vi "load station config.vi"(8 "error in":errorcluster, 11 "station config file path":path=path "c:/Labview Code/System/station config.ini") -> (0 "error out":errorcluster, 2 "Line Name":string="TP10 - All Stations Status", 3 "all satation cluster":T1[](array[typedef]) {"LIN INFO"."NAD" format="%.0x"; "LIN INFO"."ADCS LIN"."HW select" items=["NI-XNET", "NI-CAN"]; "LVDT Status"."LVDT's stored config"."Lower Limit" format="%.2f"; "LVDT Status"."LVDT's stored config"."Upper Limit" format="%.2f"; "Store Data"."Sun Shade Open Force Limits"."Variance" format="%.2g"; "Store Data"."Sun Shade Open Force Limits"."Truncation End" format="%.2g"; "Store Data"."Sun Shade Open Force Limits"."Truncation Start" format="%.2g"; "Store Data"."Sun Shade Open Force Limits"."Avg Max" format="%.2g"; "Store Data"."Sun Shade Open Force Limits"."Avg Min" format="%.2g"; "Store Data"."Sun Shade Open Force Limits"."Overall Max" format="%.2g"; "Store Data"."Sun Shade Open Force Limits"."Overall Min" format="%.2g"; "Store Data"."Sun Shade Close Force Limits"."Variance" format="%.2g"; "Store Data"."Sun Shade Close Force Limits"."Truncation End" format="%.2g"; "Store Data"."Sun Shade Close Force Limits"."Truncation Start" format="%.2g"; "Store Data"."Sun Shade Close Force Limits"."Avg Max" format="%.2g"; "Store Data"."Sun Shade Close Force Limits"."Avg Min" format="%.2g"; "Store Data"."Sun Shade Close Force Limits"."Overall Max" format="%.2g"; "Store Data"."Sun Shade Close Force Limits"."Overall Min" format="%.2g"; "Store Data"."Motion Data Array"."Motion Data Limits"."LIN Msg"."Msg" format="%02x"; "Store Data"."Motion Data Array"."Motion Data Limits"."LIN Msg"."ID" format="%02x"})   [LabVIEW 2018]
uses:
  02.Type Def's/main state cluster.ctl
  02.Type Def's/All Switch Configuration Cluster.ctl
  02.Type Def's/All Motions.ctl
  02.Type Def's/EOL Switch Value Configuration Cluster.ctl
  02.Type Def's/EOL Switch Max Min Check Cluster.ctl
  02.Type Def's/station nvh config.ctl
  02.Type Def's/station rs232 port map.ctl
  02.Type Def's/station ethernet address map.ctl
  02.Type Def's/station paths.ctl
  02.Type Def's/EOL Save Module Test Data Control.ctl
  02.Type Def's/EOL Motion Database Table.ctl
  05.UserVI's/type defs/17x Audit Motion Data Seq Control.ctl
  05.UserVI's/type defs/17x AP Data Type.ctl
  05.UserVI's/type defs/17x Sunshade Limts Seq.ctl
  02.Type Def's/EOL Module Info Control.ctl
  02.Type Def's/station DI map.ctl
  05.UserVI's/type defs/EOL Global Digital Input Control.ctl
  02.Type Def's/control refs.ctl
  02.Type Def's/station motion data indicator.ctl
  02.Type Def's/Screen Motion Data.ctl
  02.Type Def's/Pass Fail Control.ctl
  02.Type Def's/station hmi.ctl
  02.Type Def's/lvdt name val pair.ctl
  02.Type Def's/individual station status.ctl
  02.Type Def's/misc station config.ctl
  05.UserVI's/Lambda Power/power supply types.ctl
  05.UserVI's/type defs/EOL LVDT's Check Controller.ctl
  05.UserVI's/LVDT's/lvdt precision.ctl
  02.Type Def's/sequence state.ctl
  05.UserVI's/sequence/type defs/Sequence Info.ctl
  05.UserVI's/type defs/EOL Part Setup.ctl
  02.Type Def's/All Communication Types.ctl
  05.UserVI's/type defs/Communication with Motors.ctl
  05.UserVI's/type defs/RAP Signal Control.ctl
  05.UserVI's/type defs/EOL Motor Type.ctl
  02.Type Def's/station LIN config.ctl
  03.Inalfa LIN/LIN Device.ctl
  <vilib>/CMC.AME/Inalfa ADCS/Ctl'Def/ADCS_LIN info.ctl
  C:/Program Files (x86)/National Instruments/LabVIEW 2018/vi.lib/CMC.AME/Inalfa TS LIN/TOSUN/TSMaster/bin/Interop.TSMasterAPI.dll
  Program Files (x86)/National Instruments/LabVIEW 2018/vi.lib/CMC.AME/Inalfa TS LIN/TOSUN/TSMaster/bin/Interop.TSMasterAPI.dll
  06.Test Loop/Sub'VIs/Type Def's/Config Info.ctl
  05.UserVI's/file io/ini/type defs/ini entry.ctl
  05.UserVI's/file io/ini/type defs/ini entry types.ctl
  05.UserVI's/file io/ini/type defs/ini entry value.ctl
  05.UserVI's/file io/ini/type defs/ini file actions.ctl
panel:
  # "Sunroof Barcode"
  # "Pallet Number"
  # "Part Type"
  # "Application Status"
  # "Current Step"
  # "Cycle Time"
  # "Pass / Fail"
  # "Shade Close"
  # "Actual Data"
  # "Limits"
  # "Avg Current"
  # "Run Time"
  # "Speed"
  # "Noise Test"
  # "Position"
  # "Shade Open"
  # "Actual Data"
  # "Limits"
  # "Avg Current"
  # "Run Time"
  # "Speed"
  # "Noise Test"
  # "Position"
  # "Vent Close"
  # "Actual Data"
  # "Limits"
  # "Avg Current"
  # "Run Time"
  # "Speed"
  # "Noise Test"
  # "Position"
  # "Vent Open"
  # "Actual Data"
  # "Limits"
  # "Avg Current"
  # "Run Time"
  # "Speed"
  # "Noise Test"
  # "Position"
  # "Slide Close"
  # "Actual Data"
  # "Limits"
  # "Avg Current"
  # "Run Time"
  # "Speed"
  # "Noise Test"
  # "Position"
  # "Slide Open"
  # "Actual Data"
  # "Limits"
  # "Avg Current"
  # "Run Time"
  # "Speed"
  # "Noise Test"
  # "Position"
  # "Min"
  # "N"
  # "Min"
  # "Start"
  # "N"
  # "Max"
  # "N"
  # "Max"
  # "N"
  # "End"
  # "Min"
  # "N"
  # "Min"
  # "Start"
  # "N"
  # "Max"
  # "N"
  # "Max"
  # "N"
  # "End"
  # "Min"
  # "Max"
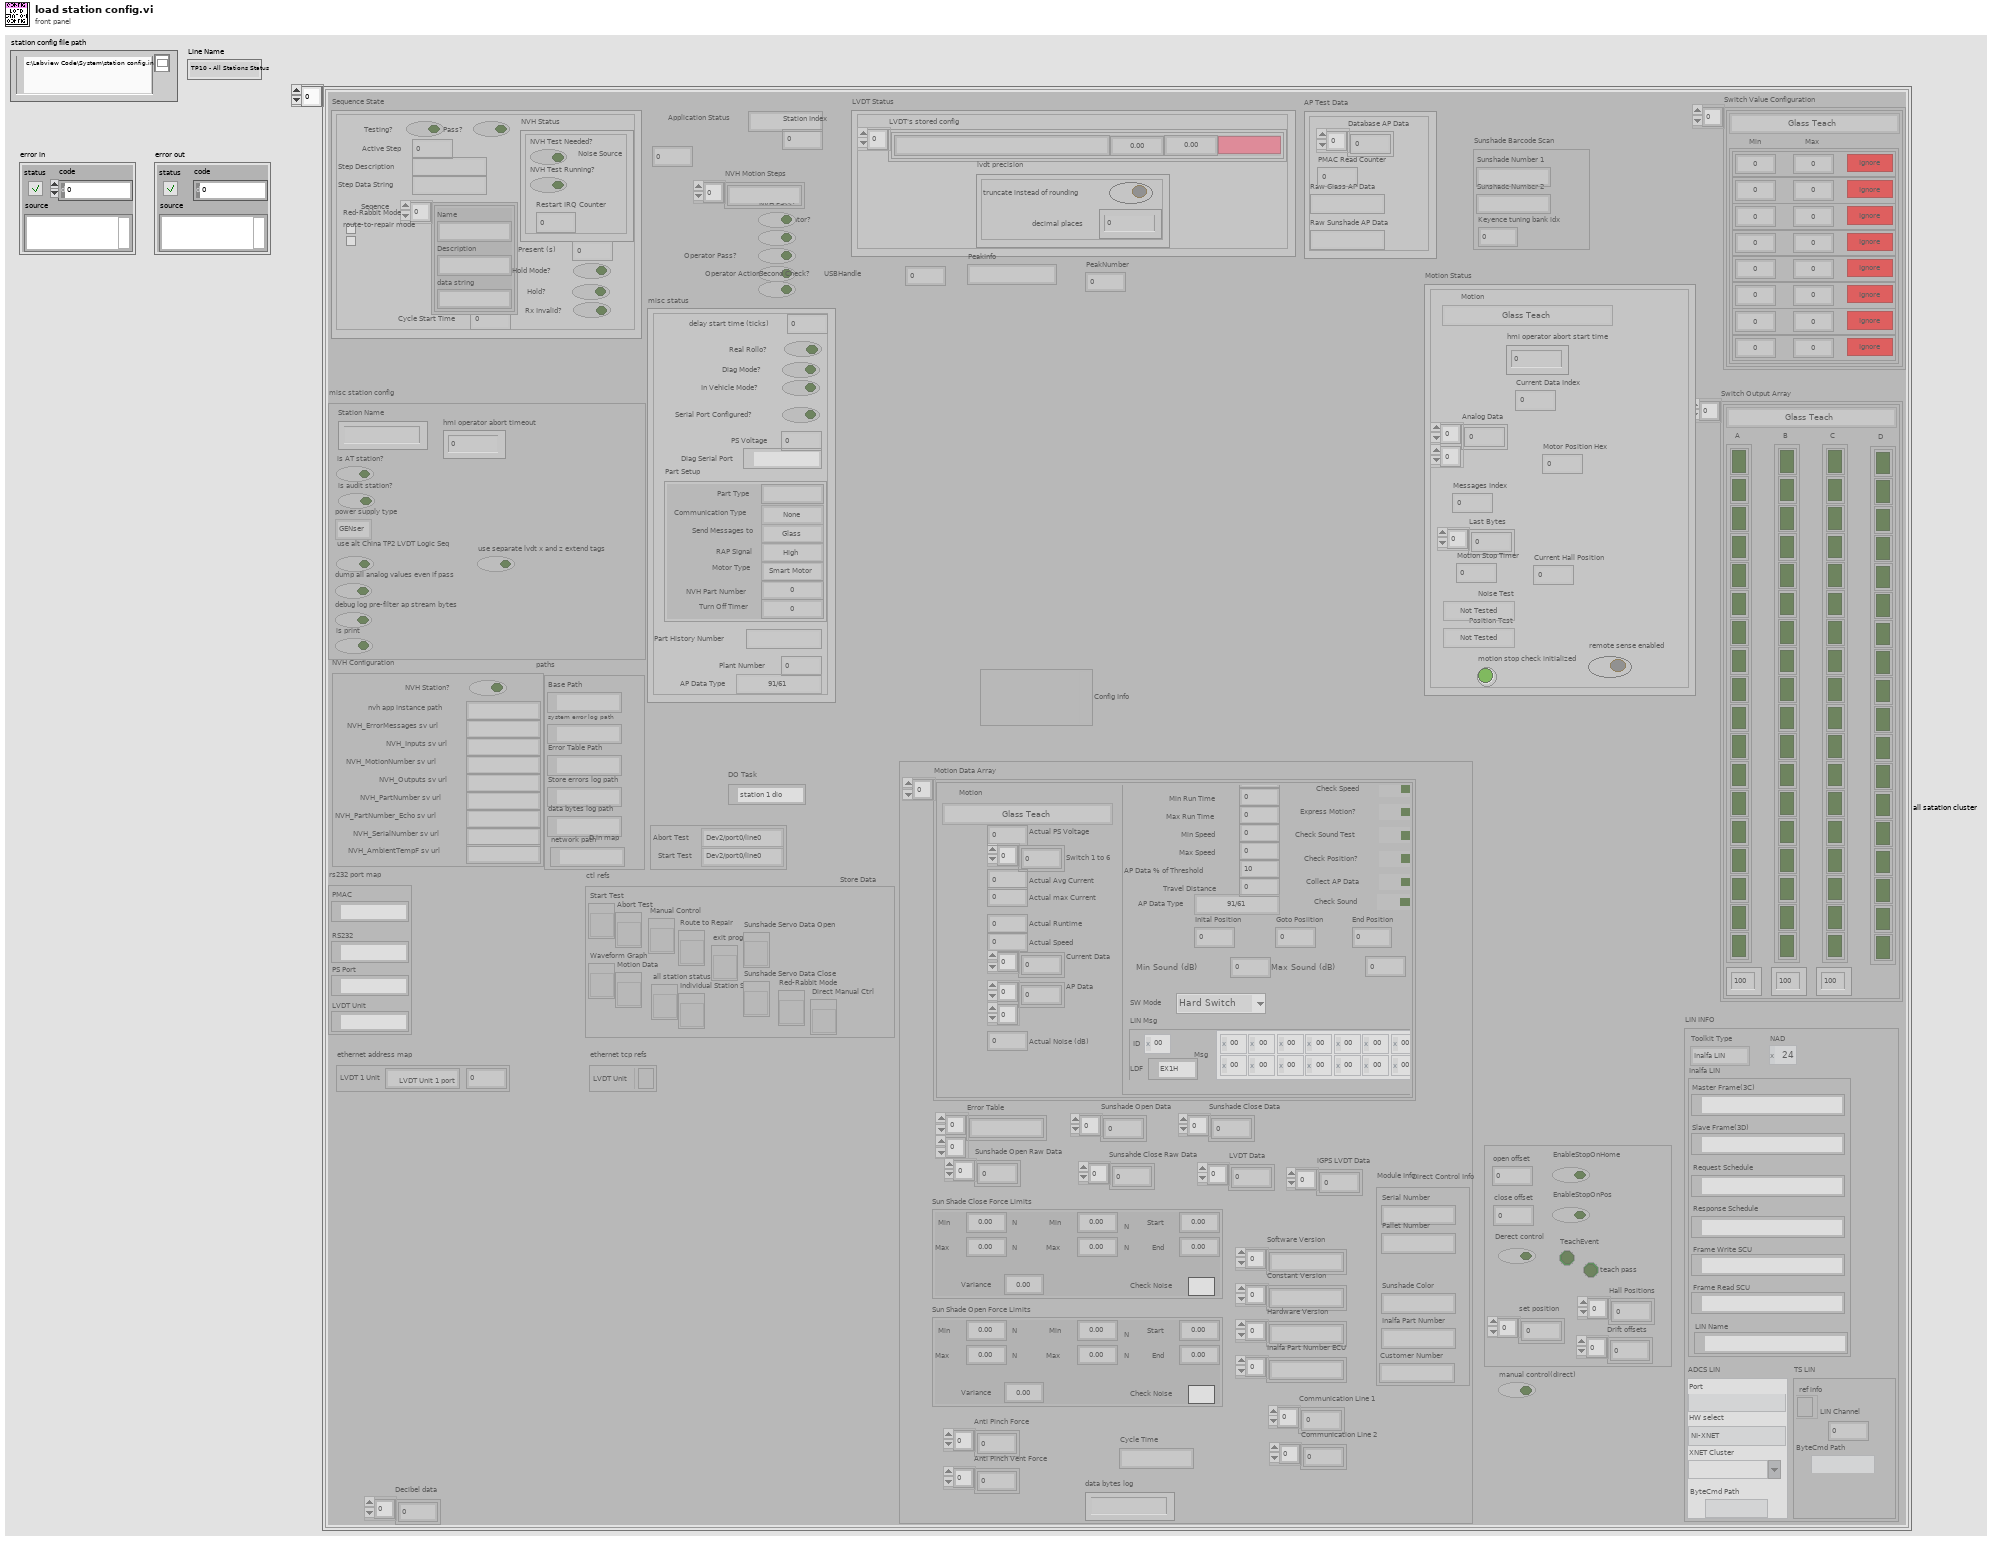
[diagram p1: front panel]
types:
  T1 = typedef "main state cluster.ctl" = cluster{"Application Status":string, "Switch Output Array":T2[], "Switch Value Configuration":T4[], "NVH Configuration":T6, "rs232 port map":T7, "ethernet address map":T8, "paths":T9, "Station Index":i32, "Store Data":T10, "D in map":T16, "DO Task":refnum<k21>, "ctl refs":T18, "misc station config":T19, "ethernet tcp refs":cluster{"LVDT Unit":refnum<k5>}, "Sunshade Barcode Scan":cluster{"Sunshade Number 2":string, "Sunshade Number 1":string, "Keyence tuning bank idx":i32}, "AP Test Data":cluster{"Raw Sunshade AP Data":string, "Raw Glass AP Data":string, "PMAC Read Counter":dbl, "Database AP Data":dbl[]}, "Motion Status":cluster{"hmi operator abort start time":u32, "Current Data Index":i32, "Analog Data":sgl[][], "Motor Position Hex":u16, "Messages Index":u16, "Last Bytes":u8[], "Current Hall Position":i16, "Motion Stop Timer":u32, "Position Test":T21, "Noise Test":T21, "motion stop check initialized":bool, "remote sense enabled":bool, "Motion":T3}, "LVDT Status":cluster{"LVDT's stored config":T22[], "lvdt precision":T23}, "Sequence State":T24, "misc status":cluster{"delay start time (ticks)":u32, "In Vehicle Mode?":bool, "Diag Mode?":bool, "Serial Port Configured?":bool, "PS Voltage":dbl, "Diag Serial Port":refnum<visa-resource-name>, "Part Setup":T26, "Part History Number":string, "Plant Number":u8, "AP Data Type":T13, "Real Rollo?":bool}, "NVH Operator?":bool, "NVH Pass?":bool, "Operator Pass?":bool, "Operator Action?":bool, "Noise Source":u32, "USBHandle":i32, "PeakInfo":string, "PeakNumber":i32, "NVH Motion Steps":string[], "Second Check?":bool, "Decibel data":dbl[], "Direct Control Info":cluster{"EnableStopOnHome":bool, "EnableStopOnPos":bool, "TeachEvent":bool, "open offset":i32, "close offset":i32, "Derect control":bool, "set position":i32[], "teach pass ":bool, "Drift offsets":i32[], "Hall Positions":i32[]}, "manual control(direct)":bool, "LIN INFO":T31, "Config Info":T34}
  T2 = typedef "All Switch Configuration Cluster.ctl" = cluster{"All Motions":T3, "A":bool[], "B":bool[], "C":bool[], "D":bool[], "A activation time (ms)":u32, "B activation time (ms)":u32, "C activation time (ms)":u32}
  T3 = typedef "All Motions.ctl" = enum16{"Glass Teach", "Glass Slide Open", "Glass Slide Close", "Glass Vent Open", "Glass Vent Close", "Sunshade Teach", "Sunshade Open", "Sunshade Close", "Idle", "Sunshade Open 2", "Sunshade Close 2", "Glass Slide Open Sunshade Open", "Glass Slide Open Sunshade Close", "Glass Slide Close Sunshade Open", "Glass Slide Close Sunshade Close", "Glass Vent Open Sunshade Open", "Glass Vent Open Sunshade Close", "Glass Vent Close Sunshade Open", "Glass Vent Close Sunshade Close", "Express Glass Slide Open", "Express Glass Slide Close", "Express Glass Vent Open", "Express Glass Vent Close", "Express Sunshade Open", "Express Sunshade Close", "Express Sunshade Open 2", "Express Sunshade Close 2", "Express Glass Slide Open Sunshade Open", "Express Glass Slide Open Sunshade Close", "Express Glass Slide Close Sunshade Open", "Express Glass Slide Close Sunshade Close", "Express Glass Vent Open Sunshade Open", "Express Glass Vent Open Sunshade Close", "Express Glass Vent Close Sunshade Open", "Express Glass Vent Close Sunshade Close", "Goto Position Glass", "Goto Position Sunshade", "Sunshade Teach 2"}
  T4 = typedef "EOL Switch Value Configuration Cluster.ctl" = cluster{"All Motions":T3, "Array":T5[]}
  T5 = typedef "EOL Switch Max Min Check Cluster.ctl" = cluster{"Min":dbl, "Max":dbl, "Check?":bool}
  T6 = typedef "station nvh config.ctl" = cluster{"NVH Station?":bool, "nvh app instance path":string, "NVH_ErrorMessages sv url":string, "NVH_Inputs sv url":string, "NVH_MotionNumber sv url":string, "NVH_Outputs sv url":string, "NVH_PartNumber sv url":string, "NVH_PartNumber_Echo sv url":string, "NVH_SerialNumber sv url":string, "NVH_AmbientTempF sv url":string}
  T7 = typedef "station rs232 port map.ctl" = cluster{"PMAC":refnum<visa-resource-name>, "PS Port":refnum<visa-resource-name>, "LVDT Unit":refnum<visa-resource-name>, "RS232":refnum<visa-resource-name>}
  T8 = typedef "station ethernet address map.ctl" = cluster{"LVDT 1 Unit":string, "LVDT Unit 1 port":u16}
  T9 = typedef "station paths.ctl" = cluster{"Base Path":path, "system error log path":path, "Error Table Path":path, "Store errors log path":path, "data bytes log path":path, "network path":path}
  T10 = typedef "EOL Save Module Test Data Control.ctl" = cluster{"Motion Data Array":T11[], "Error Table":string[][], "Sun Shade Close Force Limits":T14, "Sun Shade Open Force Limits":T14, "Sunshade Open Data":sgl[], "Sunshade Close Data":sgl[], "Module Info":T15, "Sunsahde Close Raw Data":sgl[], "Sunshade Open Raw Data":sgl[], "Software Version":string[], "Constant Version":string[], "Hardware Version":string[], "Inalfa Part Number ECU":string[], "LVDT Data":sgl[], "Communication Line 1":sgl[], "Communication Line 2":sgl[], "Anti Pinch Force":sgl[], "Cycle Time":string, "Anti Pinch Vent Force":sgl[], "iGPS LVDT Data":sgl[], "data bytes log":string}
  T11 = typedef "EOL Motion Database Table.ctl" = cluster{"Motion":T3, "Actual Avg Current":dbl, "Actual Runtime":dbl, "Actual Speed":dbl, "Current Data":sgl[], "Motion Data Limits":T12, "Switch 1 to 6":dbl[], "Actual PS Voltage":dbl, "AP Data":i16[][], "Actual max Current":dbl, "Actual Noise (dB)":dbl}
  T12 = typedef "17x Audit Motion Data Seq Control.ctl" = cluster{"Power Supply Voltage":dbl, "Min Avg Current":dbl, "Max Avg Current":dbl, "Min Run Time":dbl, "Max Run Time":dbl, "Min Speed":dbl, "Max Speed":dbl, "AP Data % of Threshold":dbl, "Travel Distance":dbl, "AP Data Type":T13, "Check Current":bool, "Check Run Time":bool, "Check Speed":bool, "Express Motion?":bool, "Check Sound Test":bool, "Check Position?":bool, "Collect AP Data":bool, "Inital Position":u16, "End Position":u16, "Goto Posiition":u16, "Max max Current":dbl, "Min max Current":dbl, "Check max Current":bool, "Check Sound":bool, "Min Sound (dB)":dbl, "Max Sound (dB)":dbl, "SW Mode":enum16{"Hard Switch", "Uncond Frame"}, "LIN Msg":cluster{"ID":u8, "Msg":u8[][], "LDF":refnum<k21>}}
  T13 = typedef "17x AP Data Type.ctl" = enum16{"91/61", "92/62", "93/63", "67", "68", "6F", "71", "91 Msg", "92 Msg", "93 Msg", "94 Msg", "HiRain 91", "HiRain 92 Speed", "HiRain 92 HS", "HiRain 92", "HiRain 93", "SnT"}
  T14 = typedef "17x Sunshade Limts Seq.ctl" = cluster{"Overall Min":dbl, "Overall Max":dbl, "Avg Min":dbl, "Avg Max":dbl, "Truncation Start":dbl, "Truncation End":dbl, "Variance":dbl, "Check Noise":bool}
  T15 = typedef "EOL Module Info Control.ctl" = cluster{"Serial Number":string, "Pallet Number":string, "Sunshade Color":string, "Inalfa Part Number":string, "Customer Number":string}
  T16 = typedef "station DI map.ctl" = cluster{"Abort Test":T17, "Start Test":T17}
  T17 = typedef "EOL Global Digital Input Control.ctl" = enum16{"Dev2/port0/line0", "Dev2/port0/line1", "Dev2/port0/line2", "Dev2/port0/line3", "Dev2/port0/line4", "Dev2/port0/line5", "Dev2/port0/line6", "Dev2/port0/line7", "Dev2/port1/line0", "Dev2/port1/line1", "Dev2/port1/line2", "Dev2/port1/line3", "Dev2/port1/line4", "Dev2/port1/line5", "Dev2/port1/line6", "Dev2/port1/line7", "Dev2/port2/line0", "Dev2/port2/line1", "Dev2/port2/line2", "Dev2/port2/line3", "Dev2/port2/line4", "Dev2/port2/line5", "Dev2/port2/line6", "Dev2/port2/line7", "Prerun Start Test", "Prerun Abort Test", "Audit Start Test", "Audit Abort Test", "Dev2/port3/line4", "Dev2/port3/line5", "Breakin Start Test", "Breakin Abort Test", "Not Implemented"}
  T18 = typedef "control refs.ctl" = cluster{"Start Test":refnum<vi>, "Abort Test":refnum<vi>, "Manual Control":refnum<vi>, "Route to Repair":refnum<vi>, "Waveform Graph":refnum<vi>, "Motion Data":refnum<vi>, "all station status":refnum<vi>, "Individual Station Status":refnum<vi>, "exit program":refnum<vi>, "Sunshade Servo Data Open":refnum<vi>, "Sunshade Servo Data Close":refnum<vi>, "Red-Rabbit Mode":refnum<vi>, "Direct Manual Ctrl":refnum<vi>}
  T19 = typedef "misc station config.ctl" = cluster{"Station Name":string, "is AT station?":bool, "is audit station?":bool, "power supply type":T20, "use alt China TP2 LVDT Logic Seq":bool, "hmi operator abort timeout":u32, "dump all analog values even if pass":bool, "debug log pre-filter ap stream bytes":bool, "use separate lvdt x and z extend tags":bool, "is print":bool}
  T20 = typedef "power supply types.ctl" = enum16{"GENser", "ZUPser", "GENeth", "Manual", "ITECH"}
  T21 = typedef "Pass Fail Control.ctl" = enum16{"Not Tested", "Pass", "Fail"}
  T22 = typedef "EOL LVDT's Check Controller.ctl" = cluster{"Upper Limit":dbl, "Lower Limit":dbl, "LVDT Name":string, "Check":bool}
  T23 = typedef "lvdt precision.ctl" = cluster{"truncate instead of rounding":bool, "decimal places":u8}
  T24 = typedef "sequence state.ctl" = cluster{"Step Description":string, "Cycle Start Time":u32, "Step Data String":string, "Pass?":bool, "Seqence":T25[], "Active Step":u8, "Testing?":bool, "Red-Rabbit Mode":bool, "route-to-repair mode":bool, "NVH Status":cluster{"Restart IRQ Counter":u8, "NVH Test Needed?":bool, "NVH Test Running?":bool}, "Present (s)":dbl, "Hold Mode?":bool, "Hold?":bool, "Rx Invalid?":bool}
  T25 = typedef "Sequence Info.ctl" = cluster{"Name":string, "Description":string, "data string":string}
  T26 = typedef "EOL Part Setup.ctl" = cluster{"Communication Type":T27, "Send Messages to":T28, "RAP Signal":T29, "Motor Type":T30, "NVH Part Number":u16, "Turn Off Timer":u16, "Part Type":string}
  T27 = typedef "All Communication Types.ctl" = enum16{"None", "CAN", "RS 232", "RS 232 LIN", "GM LIN", "SnT LIN", "K Line", "Robel CAN", "P42M-Continental", "Inalfa SCU LIN", "Spare 3"}
  T28 = typedef "Communication with Motors.ctl" = enum16{"Glass", "Rollo", "Both"}
  T29 = typedef "RAP Signal Control.ctl" = enum16{"High", "Low", "None"}
  T30 = typedef "EOL Motor Type.ctl" = enum16{"Smart Motor", "Sensor Motor"}
  T31 = typedef "station LIN config.ctl" = cluster{"Toolkit Type":enum16{"Inalfa LIN", "ADCS LIN", "TS LIN"}, "NAD":u8, "Inalfa LIN":T32, "ADCS LIN":T33, "TS LIN":cluster{"ref info":refnum<k24>, "LIN Channel":i32, "ByteCmd Path":path}}
  T32 = typedef "LIN Device.ctl" = cluster{"Master Frame(3C)":refnum<k21>, "Slave Frame(3D)":refnum<k21>, "Request Schedule":refnum<k21>, "Response Schedule":refnum<k21>, "Frame Write SCU":refnum<k21>, "Frame Read SCU":refnum<k21>, "LIN Name":refnum<k21>}
  T33 = typedef "ADCS_LIN info.ctl" = cluster{"Port":string, "HW select":u16, "XNET Cluster":string, "ByteCmd Path":path}
  T34 = typedef "Config Info.ctl" = variant
  T35 = typedef "ini file actions.ctl" = enum16{"read ini", "write ini"}
  T36 = typedef "ini entry.ctl" = cluster{"section":string, "key":string, "type":T37, "default value":T38}
  T37 = typedef "ini entry types.ctl" = enum16{"Boolean", "Double", "I32", "Path", "String", "U32"}
  T38 = typedef "ini entry value.ctl" = cluster{"Boolean":bool, "Dbl":dbl, "I32":i32, "Path":path, "String":string, "U32":u32}
  T39 = typedef "plc comms params.ctl" = cluster{"PLC boolean read Tags":T40, "PLC bool write Tags":T43, "PLC string read Tags":T44, "PLC string write Tags":T45, "use opc":bool, "PLC/OPC Path":string}
  T40 = typedef "station plc read boolean tags.ctl" = cluster{"AT glass position":T41, "AT shade position":T41, "AT in glass wand lower pos":T41, "AT in glass wand up pos":T41, "AT in sunshad wand lower pos":T41, "AT in sunshad wand up pos":T41, "AT in wand home pos":T41, "LVDT's Extended":T41, "bolt check 1":T41, "bolt check 2":T41, "bolt check 3":T41, "bolt check 4":T41, "bolt check 5":T41, "bolt check 6":T41, "bolt check 7":T41, "bolt check 8":T41, "start":T41, "abort":T41, "LVDT's Retracted":T41, "manual barcode print":T41, "ss servo at open":T41, "ss servo at close":T41, "ss servo opening":T41, "ss servo closing":T41, "control slide at home":T41, "control slide left good":T41, "control slide left over stroke":T41, "control slide right good":T41, "control slide right over stroke":T41, "wind deflector high speed pos":T41, "wind deflector low speed pos":T41, "AT VentPMACatHome":T41, "AT VentPMACisExtend":T41, "SS Barcode Scanner Bypassed":T41, "Check Frame Barcode":T41, "Z LVDTs Extended":T41, "NVH Operator Pass":T41, "NVH Operator Fail":T41, "NVH Operator Express Glass Open":T41, "NVH Operator Express Glass Close":T41, "NVH Operator Express Rollo Open01":T41, "NVH Operator Express Rollo Close01":T41, "NVH Operator Express Rollo Open02":T41, "NVH Operator Express Rollo Close02":T41, "NVH Operator Vent Open Noise":T41, "NVH Operator Vent Close Noise":T41, "NVH Operator Sunshade Open Noise":T41, "NVH Operator Sunshade Close Noise":T41, "NVH Operator Glass Open Noise":T41, "NVH Operator Glass Close Noise":T41, "NVH Operator Finish":T41, "NVH Operator Check":T41, "windproof position":T41, "NVH Operator Express Glass vent Open":T41, "NVH Operator Express Glass Vent Close":T41, "NVH Operator Re-do":T41, "AT at vent ATS test pos":T41, "AT at vent ATS Home pos":T41, "Start Adjust LVDT":T41, "Finish Adjust LVDT":T41}
  T41 = typedef "plc path and tag.ctl" = cluster{"Tag Name":string, "Network Path":string, "use opc":bool, "DataSocket Reference":T42}
  T42 = typedef "DataSocket Reference Type.ctl" = cluster{"CWDSLib._DCWDataSocket":refnum<k7>, "CWDSLib._DCWData":refnum<k7>, "OnDataUpdated":u32, "OnStatusUpdated":u32}
  T43 = typedef "station plc write boolean tags.ctl" = cluster{"AT set glass wand lower":T41, "AT set sunshade wand lower":T41, "AT set sunshade wand up":T41, "AT set glass wand up":T41, "AT set wand home pos":T41, "Test Complete Pass":T41, "Test Complete Fail":T41, "Test Started":T41, "Retract LVDT's":T41, "Extend LVDT's":T41, "ss servo open":T41, "ss servo close":T41, "control slide start":T41, "control slide stop":T41, "AT VentPMACHome":T41, "AT VentPMACExtended":T41, "Good Frame Barcode":T41, "Bad Frame Barcode":T41, "Extend Z LVDTS":T41, "NVH SunRoof Moving":T41, "NVH SunRoof Stop":T41, "NVH Pass":T41, "NVH Fail":T41, "NVH Operator Express Glass Opened":T41, "NVH Operator Express Glass Closed":T41, "NVH Operator Express Rollo Opened01":T41, "NVH Operator Express Rollo Closed01":T41, "NVH Operator Express Rollo Opened02":T41, "NVH Operator Pass":T41, "NVH Operator Fail":T41, "NVH Operator Check":T41, "NVH Operator Vent Open Noise":T41, "NVH Operator Vent Close Noise":T41, "NVH Operator Sunshade Open Noise":T41, "NVH Operator Sunshade Close Noise":T41, "NVH Operator Glass Open Noise":T41, "NVH Operator Glass Close Noise":T41, "NVH Operator Finish":T41, "Barcode01 OK":T41, "Barcode02 OK":T41, "AT set to Vent ATS Test Pos":T41, "AT set to Vent ATS Home Pos":T41, "Move LVDT Adjust Station":T41}
  T44 = typedef "station plc read string tags.ctl" = cluster{"Serial Number":T41, "Pallet Number":T41, "Inalfa Part Number":T41, "Shade Color":T41, "Model Type":T41, "Customer Number":T41, "Part History Number":T41, "Shade 1 Barcode":T41, "Shade 2 Barcode":T41, "Manual Serial Number":T41, "Manual Inalfa Part Number":T41, "Manual Shade Color":T41, "Manual Model Type":T41, "Manual Customer Number":T41, "Manual Part History Number":T41}
  T45 = typedef "station plc write string tags.ctl" = cluster{"barcode station error":T41, "error message 0":T41, "error message 1":T41, "error message 2":T41, "error message 3":T41}
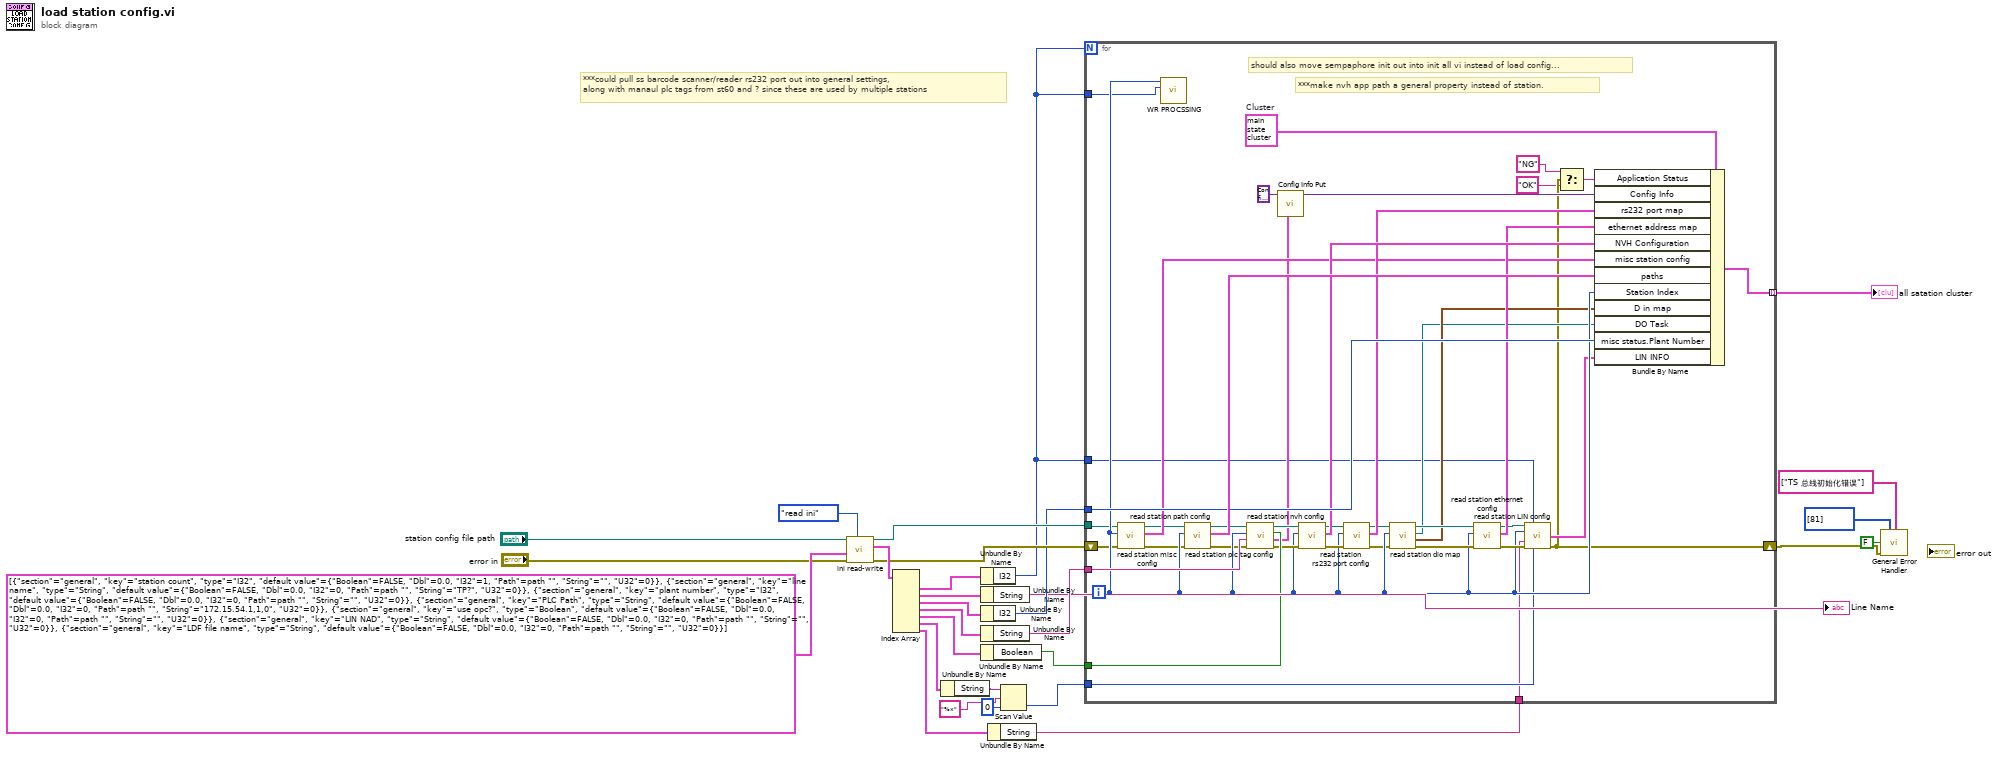
[diagram p0: block diagram]
diagram:
  # "***could pull ss barcode scanner/reader rs232 port out into general settings,\nalong with manaul plc tags from st60 and ? since these are used by multiple stations"
  n1 = call "ini read-write.vi"("action"=ini_file_actions."read ini", "error in (no error)"="error in", "ini entry descriptors"=T36[] [{"section"="general", "key"="station count", "type"=enum."I32", "default value"={"Boolean"=FALSE, "Dbl"=0.0, "I32"=1, "Path"=path "", "String"="", "U32"=0}}, {"section"="general", "key"="line name", "type"=enum."String", "default value"={"Boolean"=FALSE, "Dbl"=0.0, "I32"=0, "Path"=path "", "String"="TP?", "U32"=0}}, {"section"="general", "key"="plant number", "type"=enum."I32", "default value"={"Boolean"=FALSE, "Dbl"=0.0, "I32"=0, "Path"=path "", "String"="", "U32"=0}}, {"section"="general", "key"="PLC Path", "type"=enum."String", "default value"={"Boolean"=FALSE, "Dbl"=0.0, "I32"=0, "Path"=path "", "String"="172.15.54.1,1,0", "U32"=0}}, {"section"="general", "key"="use opc?", "type"=enum."Boolean", "default value"={"Boolean"=FALSE, "Dbl"=0.0, "I32"=0, "Path"=path "", "String"="", "U32"=0}}, {"section"="general", "key"="LIN NAD", "type"=enum."String", "default value"={"Boolean"=FALSE, "Dbl"=0.0, "I32"=0, "Path"=path "", "String"="", "U32"=0}}, {"section"="general", "key"="LDF file name", "type"=enum."String", "default value"={"Boolean"=FALSE, "Dbl"=0.0, "I32"=0, "Path"=path "", "String"="", "U32"=0}}], "configuration file path"="station config file path") -> ("error out"=w22:errorcluster, "values out"=w27:T38[], "configuration file path out"=w24:path)  [unwired: 5 in]
  n2 = Index Array(array=w27) -> (element #1=w26:T38, element #2=w25:T38, element #3=w21:T38, element #4=w19:T38, element #5=w17:T38, element #6=w7:T38, element #7=w6:T38)  [unwired: 7 in]
  n3 = Unbundle By Name(w7) -> ("String"=w11:string)
  n4 = Unbundle By Name(w26) -> ("I32"=w8:i32)
  n5 = Unbundle By Name(w25) -> ("String"=→"Line Name":string)
  n6 = Unbundle By Name(w21) -> ("I32"=w20:i32)
  n7 = Unbundle By Name(w19) -> ("String"=w18:string)
  n8 = Unbundle By Name(w17) -> ("Boolean"=w16:bool)
  n9 = Unbundle By Name(w6) -> ("String"=w9:string)
  n10 = Scan Value(string=w11, format string="%x" ("格式字符串"), default (0 dbl)=u8 0 ("NAD")) -> (value=w10:u8)  [unwired: 1 out]
  n11 = for {
    N: w8 -> [_]
    tunnel: [w70] -> w14 mode=indexing
    tunnel: w24 -> [w36]
    shift-right: [w33] -> w2
    shift-left: w22 -> [w37]
    tunnel: w20 -> [w68]
    tunnel: w18 -> [w63]
    tunnel: w16 -> [w64]
    tunnel: w8 -> [w42]
    tunnel: w10 -> [w48]
    tunnel: w9 -> [w47]
    tunnel: w8 -> [w40]
    i -> [w54]
    w50 = T1 {"Application Status"="", "Switch Output Array"=[], "Switch Value Configuration"=[], "NVH Configuration"={"NVH Station?"=FALSE, "nvh app instance path"="", "NVH_ErrorMessages sv url"="", "NVH_Inputs sv url"="", "NVH_MotionNumber sv url"="", "NVH_Outputs sv url"="", "NVH_PartNumber sv url"="", "NVH_PartNumber_Echo sv url"="", "NVH_SerialNumber sv url"="", "NVH_AmbientTempF sv url"=""}, "rs232 port map"={"PMAC"="COM3", "PS Port"="COM27", "LVDT Unit"="COM36", "RS232"="COM24"}, "ethernet address map"={"LVDT 1 Unit"="172.17.53.143", "LVDT Unit 1 port"=0}, "paths"={"Base Path"=path "", "system error log path"=path "", "Error Table Path"=path "C:/Labview Code/System/Error Table", "Store errors log path"=path "C:/Labview Code/System/Error Table", "data bytes log path"=path "C:/Labview Code/System/Error Table", "network path"=path "C:/Labview Code/System/Error Table"}, "Station Index"=0, "Store Data"={"Motion Data Array"=[], "Error Table"=[], "Sun Shade Close Force Limits"={"Overall Min"=0.0, "Overall Max"=0.0, "Avg Min"=0.0, "Avg Max"=0.0, "Truncation Start"=0.0, "Truncation End"=0.0, "Variance"=0.0, "Check Noise"=FALSE}, "Sun Shade Open Force Limits"={"Overall Min"=0.0, "Overall Max"=0.0, "Avg Min"=0.0, "Avg Max"=0.0, "Truncation Start"=0.0, "Truncation End"=0.0, "Variance"=0.0, "Check Noise"=FALSE}, "Sunshade Open Data"=[], "Sunshade Close Data"=[], "Module Info"={"Serial Number"="", "Pallet Number"="", "Sunshade Color"="", "Inalfa Part Number"="", "Customer Number"=""}, "Sunsahde Close Raw Data"=[], "Sunshade Open Raw Data"=[], "Software Version"=[], "Constant Version"=[], "Hardware Version"=[], "Inalfa Part Number ECU"=[], "LVDT Data"=[], "Communication Line 1"=[], "Communication Line 2"=[], "Anti Pinch Force"=[], "Cycle Time"="", "Anti Pinch Vent Force"=[], "iGPS LVDT Data"=[], "data bytes log"=""}, "D in map"={"Abort Test"=enum."Dev2/port0/line0", "Start Test"=enum."Dev2/port0/line0"}, "DO Task"="station 1 dio", "ctl refs"={"Start Test"=refnum, "Abort Test"=refnum, "Manual Control"=refnum, "Route to Repair"=refnum, "Waveform Graph"=refnum, "Motion Data"=refnum, "all station status"=refnum, "Individual Station Status"=refnum, "exit program"=refnum, "Sunshade Servo Data Open"=refnum, "Sunshade Servo Data Close"=refnum, "Red-Rabbit Mode"=refnum, "Direct Manual Ctrl"=refnum}, "misc station config"={"Station Name"="", "is AT station?"=FALSE, "is audit station?"=FALSE, "power supply type"=enum."GENser", "use alt China TP2 LVDT Logic Seq"=FALSE, "hmi operator abort timeout"=0, "dump all analog values even if pass"=FALSE, "debug log pre-filter ap stream bytes"=FALSE, "use separate lvdt x and z extend tags"=FALSE, "is print"=FALSE}, "ethernet tcp refs"={"LVDT Unit"=refnum}, "Sunshade Barcode Scan"={"Sunshade Number 2"="", "Sunshade Number 1"="", "Keyence tuning bank idx"=0}, "AP Test Data"={"Raw Sunshade AP Data"="", "Raw Glass AP Data"="", "PMAC Read Counter"=0.0, "Database AP Data"=[]}, "Motion Status"={"hmi operator abort start time"=0, "Current Data Index"=0, "Analog Data"=[], "Motor Position Hex"=0, "Messages Index"=0, "Last Bytes"=[], "Current Hall Position"=0, "Motion Stop Timer"=0, "Position Test"=enum."Not Tested", "Noise Test"=enum."Not Tested", "motion stop check initialized"=FALSE, "remote sense enabled"=FALSE, "Motion"=enum."Glass Teach"}, "LVDT Status"={"LVDT's stored config"=[{"Upper Limit"=1.0, "Lower Limit"=-1.0, "LVDT Name"="LVDT 1", "Check"=FALSE}, {"Upper Limit"=1.0, "Lower Limit"=-1.0, "LVDT Name"="LVDT 2", "Check"=FALSE}, {"Upper Limit"=1.0, "Lower Limit"=-1.0, "LVDT Name"="LVDT 3", "Check"=FALSE}, {"Upper Limit"=1.0, "Lower Limit"=-1.0, "LVDT Name"="LVDT 4", "Check"=FALSE}, {"Upper Limit"=1.0, "Lower Limit"=-1.0, "LVDT Name"="LVDT 5", "Check"=FALSE}, {"Upper Limit"=1.0, "Lower Limit"=-1.0, "LVDT Name"="LVDT 6", "Check"=FALSE}, {"Upper Limit"=1.0, "Lower Limit"=-1.0, "LVDT Name"="LVDT 7", "Check"=FALSE}, {"Upper Limit"=1.0, "Lower Limit"=-1.0, "LVDT Name"="LVDT 8", "Check"=FALSE}, {"Upper Limit"=1.0, "Lower Limit"=-1.0, "LVDT Name"="LVDT 9", "Check"=FALSE}, {"Upper Limit"=1.0, "Lower Limit"=-1.0, "LVDT Name"="LVDT 10", "Check"=FALSE}, {"Upper Limit"=1.0, "Lower Limit"=-1.0, "LVDT Name"="LVDT 11", "Check"=FALSE}, {"Upper Limit"=1.0, "Lower Limit"=-1.0, "LVDT Name"="LVDT 12", "Check"=FALSE}, {"Upper Limit"=1.0, "Lower Limit"=-1.0, "LVDT Name"="LVDT 13", "Check"=FALSE}, {"Upper Limit"=1.0, "Lower Limit"=-1.0, "LVDT Name"="LVDT 14", "Check"=FALSE}], "lvdt precision"={"truncate instead of rounding"=FALSE, "decimal places"=0}}, "Sequence State"={"Step Description"="", "Cycle Start Time"=0, "Step Data String"="", "Pass?"=FALSE, "Seqence"=[], "Active Step"=0, "Testing?"=FALSE, "Red-Rabbit Mode"=FALSE, "route-to-repair mode"=FALSE, "NVH Status"={"Restart IRQ Counter"=0, "NVH Test Needed?"=FALSE, "NVH Test Running?"=FALSE}, "Present (s)"=0.0, "Hold Mode?"=FALSE, "Hold?"=FALSE, "Rx Invalid?"=FALSE}, "misc status"={"delay start time (ticks)"=0, "In Vehicle Mode?"=FALSE, "Diag Mode?"=FALSE, "Serial Port Configured?"=FALSE, "PS Voltage"=0.0, "Diag Serial Port"="", "Part Setup"={"Communication Type"=enum."None", "Send Messages to"=enum."Glass", "RAP Signal"=enum."High", "Motor Type"=enum."Smart Motor", "NVH Part Number"=0, "Turn Off Timer"=0, "Part Type"=""}, "Part History Number"="", "Plant Number"=0, "AP Data Type"=enum."91/61", "Real Rollo?"=FALSE}, "NVH Operator?"=FALSE, "NVH Pass?"=FALSE, "Operator Pass?"=FALSE, "Operator Action?"=FALSE, "Noise Source"=0, "USBHandle"=0, "PeakInfo"="", "PeakNumber"=0, "NVH Motion Steps"=[], "Second Check?"=FALSE, "Decibel data"=[], "Direct Control Info"={"EnableStopOnHome"=FALSE, "EnableStopOnPos"=FALSE, "TeachEvent"=FALSE, "open offset"=0, "close offset"=0, "Derect control"=FALSE, "set position"=[], "teach pass "=FALSE, "Drift offsets"=[], "Hall Positions"=[]}, "manual control(direct)"=FALSE, "LIN INFO"={"Toolkit Type"=enum."Inalfa LIN", "NAD"=36, "Inalfa LIN"={"Master Frame(3C)"="", "Slave Frame(3D)"="NIXNET_exampleLDF", "Request Schedule"="NIXNET_exampleLDF", "Response Schedule"="CEMLIN3DiagResponseSchedule\nSPA3414_ConfigurationsCMAGeely_CEMCALYPSOSDB34XX0Cfg_LIN3_190709_", "Frame Write SCU"="", "Frame Read SCU"="", "LIN Name"=""}, "ADCS LIN"={"Port"="MasterReq\nSPA3414_ConfigurationsCMAGeely_CEMCALYPSOSDB34XX0Cfg_LIN3_190709_", "HW select"=0, "XNET Cluster"="SlaveResp\nSPA3414_ConfigurationsCMAGeely_CEMCALYPSOSDB34XX0Cfg_LIN3_190709_", "ByteCmd Path"=path "C:/Labview Code/System/ByteCmdConfig.txt"}, "TS LIN"={"ref info"=refnum, "LIN Channel"=0, "ByteCmd Path"=path "C:/Labview Code/System/ByteCmdConfig.txt"}}, "Config Info"=variant}  # Cluster
    # "***make nvh app path a general property instead of station."
    # "should also move sempaphore init out into init all vi instead of load config..."
    n12 = call "read station misc config.vi"("error in"=w37, "station idx"=w54, "configuration file path in"=w36) -> ("error out"=w38:errorcluster, "misc station config"=w53:T19, "configuration file path out"=w35:path)  [unwired: 6 in]
    n13 = call "WR PROCSSING.vi"("标尺.范围:最大值"=w42, "进度"=w54) -> ()  [unwired: 9 in, 1 out]
    n14 = call "read station path config.vi"("error in"=w38, "station idx"=w54, "configuration file path in"=w35) -> ("error out"=w39:errorcluster, "paths"=w69:T9, "configuration file path out"=w34:path)  [unwired: 6 in]
    n15 = call "read station plc tag config.vi"("use opc"=w64, "error in"=w39, "PLC Path"=w63, "station idx"=w54, "configuration file path in"=w34) -> ("error out"=w57:errorcluster, "PLC Comms"=w41:T39, "configuration file path out"=w58:path)  [unwired: 3 in, 1 out]
    n16 = call "Config Info Put.vi"("PLC Comms"=w41, "Config Info"=T34 variant) -> ("Config Info out"=w44:T34)  [unwired: 8 in, 1 out]
    n17 = call "read station nvh config.vi"("error in"=w57, "station idx"=w54, "configuration file path in"=w58) -> ("error out"=w61:errorcluster, "st nvh config"=w67:T6, "configuration file path out"=w62:path)  [unwired: 6 in]
    n18 = call "read station rs232 port config.vi"("error in"=w61, "station idx"=w54, "configuration file path in"=w62) -> ("error out"=w52:errorcluster, "rs232 port map"=w66:T7, "configuration file path out"=w51:path)  [unwired: 6 in]
    n19 = call "read station dio map.vi"("error in"=w52, "station idx"=w54, "configuration file path in"=w51) -> ("error out"=w59:errorcluster, "D in map"=w46:T16, "DO Task"=w43:refnum<k21>, "configuration file path out"=w60:path)  [unwired: 4 in]
    n20 = call "read station ethernet config.vi"("error in"=w59, "station idx"=w54, "configuration file path in"=w60) -> ("error out"=w55:errorcluster, "ethernet address map"=w65:T8, "configuration file path out"=w56:path)  [unwired: 6 in]
    n21 = call "read station LIN config.vi"("configuration file path in"=w56, "lin channel count"=w40, "station idx"=w54, "ldf file name"=w47, "error in"=w55, "NAD"=w48) -> ("LIN INFO"=w49:T31, "error out"=w33:errorcluster)  [unwired: 6 in, 2 out]
    n22 = Select(t="NG", s=w33, f="OK") -> (s? t:f=w30:string)
    n23 = Bundle By Name(cluster=w50, "Application Status"=w30, "Config Info"=w44, "rs232 port map"=w66, "ethernet address map"=w65, "NVH Configuration"=w67, "misc station config"=w53, "paths"=w69, "Station Index"=w54, "D in map"=w46, "DO Task"=w43, "misc status.Plant Number"=w68, "LIN INFO"=w49) -> (w70:T1)
  }
  "all satation cluster" <- w14
  n24 = call <vilib>:"General Error Handler.vi"("[user-defined codes]"=i32[] [81], "[user-defined descriptions]"=string[] ["TS 总线初始化错误"], "search ni.com link visible?(T)"=FALSE, "error in (no error)"=w2) -> ()  [unwired: 7 in, 5 out]
